vi "SCLN_CloseServers.vi"(0 "Server Name":string) -> ()   [LabVIEW 2015]
uses:
  SCLN_RW_Select.ctl
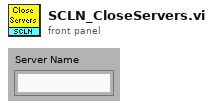
[diagram p1: front panel]
types:
  T1 = typedef "SCLN_RW_Select.ctl" = enum16{"Read", "Write"}
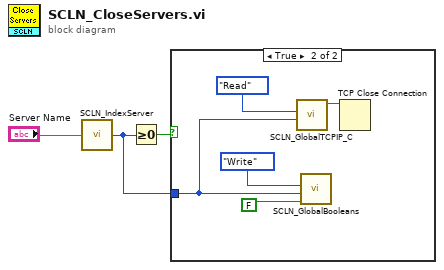
[diagram p0: block diagram]
diagram:
  n1 = call "SCLN_IndexServer.vi"("Server Name"="Server Name") -> ("Index"=w1:i32)
  n2 = Greater Or Equal To 0?(x=w1) -> (x >= 0?=w2:bool)
  n3 = case shown="True" w2 {
    tunnel: w1 -> [_ w6]
    frame False {
    }
    frame True {
      n4 = call "SCLN_GlobalTCPIP_C.vi"("Element"=w6, "Operation"=SCLN_RW_Select."Read" ("GBL_RW")) -> ("TCPIP_Id Read"=w4:refnum<k5>)  [unwired: 2 in, 1 out]
      n5 = call "SCLN_GlobalBooleans.vi"("Write Value"=FALSE, "Element"=w6, "Operation"=SCLN_RW_Select."Write" ("GBL_RW")) -> ()  [unwired: 1 in, 2 out]
      n6 = TCP Close Connection(connection ID=w4) -> ()  [unwired: 2 in, 2 out]
    }
  }
